vi "LWXPS_GroupAllPositionTrace.vi"(6 "LabVIEW error IN":errorcluster, 7 "Title Trace":string, 8 "Group Name":string, 9 "XPS Reference IN":refnum<k24>) -> (0 "LabVIEW error OUT":errorcluster, 1 "XPS Error String":string, 2 "Returned error code":i32, 3 "XPS Reference OUT":refnum<k24>)   [LabVIEW 2014]
uses:
  D:/XPSQ8_LabView_Library/Development/Source/Dll/Newport.XPS.CommandInterface.dll
  Dll/Newport.XPS.CommandInterface.dll
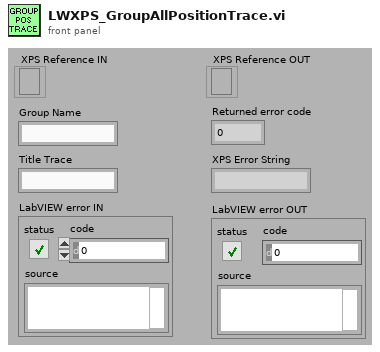
[diagram p1: front panel]
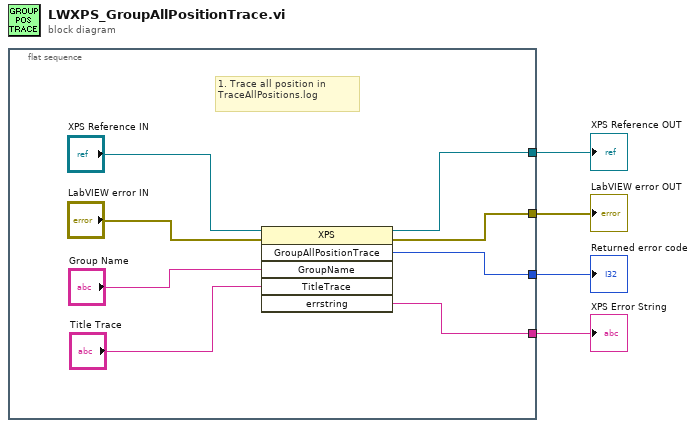
[diagram p0: block diagram]
diagram:
  n1 = flat-sequence {
    tunnel: [w9] -> w4
    tunnel: [w12] -> w3
    tunnel: [w10] -> w2
    tunnel: [w7] -> w1
    frame #0 {
      # "1. Trace all position in TraceAllPositions.log"
      n2 = invoke class="XPS" method="GroupAllPositionTrace"(reference="XPS Reference IN", error in="LabVIEW error IN", "GroupName"="Group Name", "TitleTrace"="Title Trace") -> (reference out=w9:refnum<k24>, error out=w12:errorcluster, "GroupAllPositionTrace"=w10:i32, "errstring"=w7:string)  [unwired: 2 in, 2 out]
    }
  }
  "XPS Reference OUT" <- w4
  "LabVIEW error OUT" <- w3
  "Returned error code" <- w2
  "XPS Error String" <- w1
